vi "CheckParameters.vi"(8 "error in (no error)":errorcluster, 10 "Parameters":u32[](array[numeric]), 11 "Burst in":refnum<class "Burst.lvclass">) -> (0 "error out":errorcluster, 3 "Burst out":refnum<class "Burst.lvclass">)   [LabVIEW 2013, in "Burst.lvclass"]
uses:
  Burst.lvclass
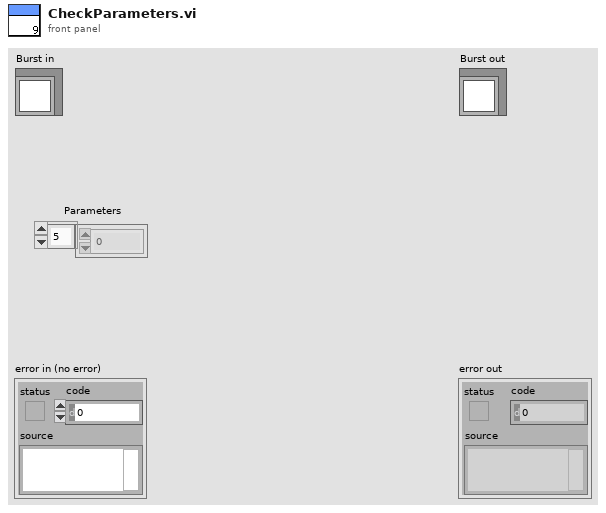
[diagram p1: front panel]
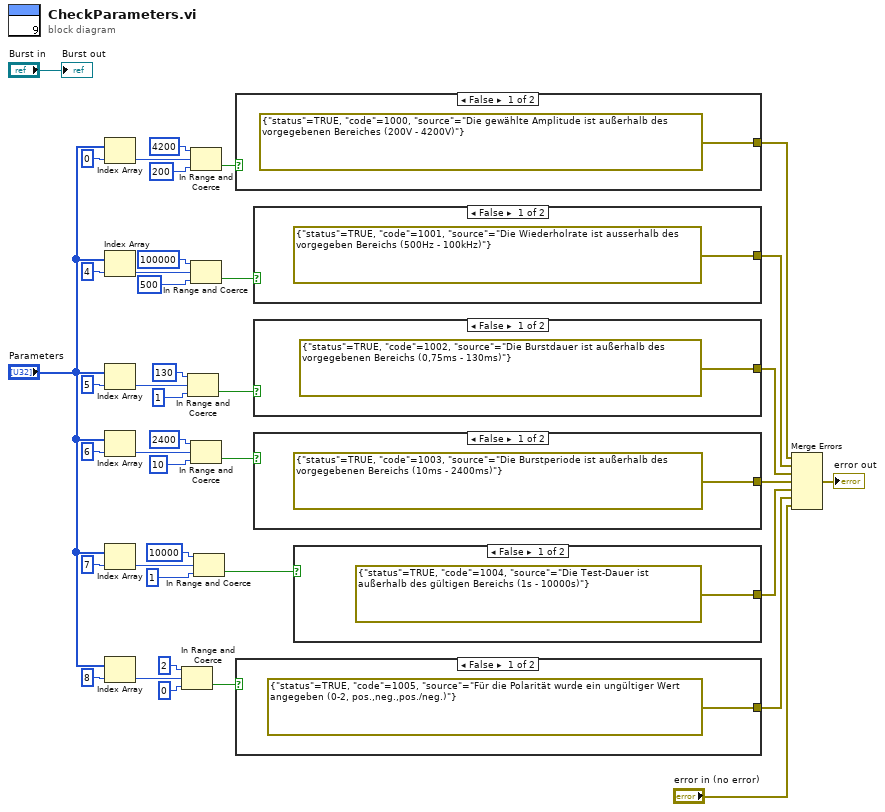
[diagram p0: block diagram]
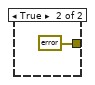
[diagram p2: hidden frame]
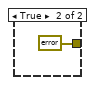
[diagram p3: hidden frame]
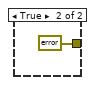
[diagram p4: hidden frame]
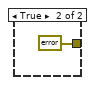
[diagram p5: hidden frame]
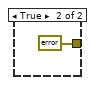
[diagram p6: hidden frame]
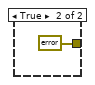
[diagram p7: hidden frame]
diagram:
  n1 = Index Array(array="Parameters", index=0) -> (element=w39:u32)
  n2 = Index Array(array="Parameters", index=4) -> (element=w33:u32)
  n3 = Index Array(array="Parameters", index=5) -> (element=w32:u32)
  n4 = Index Array(array="Parameters", index=6) -> (element=w27:u32)
  n5 = Index Array(array="Parameters", index=7) -> (element=w26:u32)
  n6 = Index Array(array="Parameters", index=8) -> (element=w15:u32)
  n7 = In Range and Coerce(upper limit=u32 2, x=w15, lower limit=u32 0) -> (In Range?=w13:bool)  [unwired: 1 out]
  n8 = In Range and Coerce(upper limit=u32 130, x=w32, lower limit=u32 1) -> (In Range?=w10:bool)  [unwired: 1 out]
  n9 = In Range and Coerce(upper limit=u32 4200, x=w39, lower limit=u32 200) -> (In Range?=w37:bool)  [unwired: 1 out]
  n10 = In Range and Coerce(upper limit=u32 100000, x=w33, lower limit=u32 500) -> (In Range?=w9:bool)  [unwired: 1 out]
  n11 = In Range and Coerce(upper limit=u32 2400, x=w27, lower limit=u32 10) -> (In Range?=w11:bool)  [unwired: 1 out]
  n12 = In Range and Coerce(upper limit=u32 10000, x=w26, lower limit=u32 1) -> (In Range?=w12:bool)  [unwired: 1 out]
  n13 = case shown="False" w37 {
    tunnel: [errorcluster {"status"=TRUE, "code"=1000, "source"="Die gewählte Amplitude ist außerhalb des vorgegebenen Bereiches (200V - 4200V)"} ("error constant") errorcluster {"status"=FALSE, "code"=0, "source"=""} ("error constant")] -> w8
    frame False {
    }
    frame True {
    }
  }
  n14 = case shown="False" w13 {
    tunnel: [errorcluster {"status"=TRUE, "code"=1005, "source"="Für die Polarität wurde ein ungültiger Wert angegeben (0-2, pos.,neg.,pos./neg.)"} ("error constant") errorcluster {"status"=FALSE, "code"=0, "source"=""} ("error constant")] -> w3
    frame False {
    }
    frame True {
    }
  }
  n15 = case shown="False" w9 {
    tunnel: [errorcluster {"status"=TRUE, "code"=1001, "source"="Die Wiederholrate ist ausserhalb des vorgegeben Bereichs (500Hz - 100kHz)"} ("error constant") errorcluster {"status"=FALSE, "code"=0, "source"=""} ("error constant")] -> w7
    frame False {
    }
    frame True {
    }
  }
  n16 = case shown="False" w10 {
    tunnel: [errorcluster {"status"=TRUE, "code"=1002, "source"="Die Burstdauer ist außerhalb des vorgegebenen Bereichs (0,75ms - 130ms)"} ("error constant") errorcluster {"status"=FALSE, "code"=0, "source"=""} ("error constant")] -> w6
    frame False {
    }
    frame True {
    }
  }
  n17 = case shown="False" w11 {
    tunnel: [errorcluster {"status"=TRUE, "code"=1003, "source"="Die Burstperiode ist außerhalb des vorgegebenen Bereichs (10ms - 2400ms)"} ("error constant") errorcluster {"status"=FALSE, "code"=0, "source"=""} ("error constant")] -> w5
    frame False {
    }
    frame True {
    }
  }
  n18 = case shown="False" w12 {
    tunnel: [errorcluster {"status"=TRUE, "code"=1004, "source"="Die Test-Dauer ist außerhalb des gültigen Bereichs (1s - 10000s)"} ("error constant") errorcluster {"status"=FALSE, "code"=0, "source"=""} ("error constant")] -> w4
    frame False {
    }
    frame True {
    }
  }
  n19 = Merge Errors(w8, w7, w6, w5, w4, w3, "error in (no error)") -> (→"error out":errorcluster)
  "Burst out" <- "Burst in"
